vi "Read Show FP.vi"(8 "error in (no error)":errorcluster, 11 "Launch Functions Message in":refnum<class "Launch Functions Message.lvclass">) -> (0 "error out":errorcluster, 2 "Show FP?":bool, 3 "Launch Functions Message out":refnum<class "Launch Functions Message.lvclass">)   [LabVIEW 2016, in "Controller Actor.lvlib" / "Launch Functions Message.lvclass"]
uses:
  <userlib>/Common Components/Controller/Messages/Launch Functions Message/Launch Functions Message.lvclass
  <userlib>/Common Components/Controller/Messages/Launch Functions Message/Launch Functions Message.lvclass/Launch Functions Message.ctl
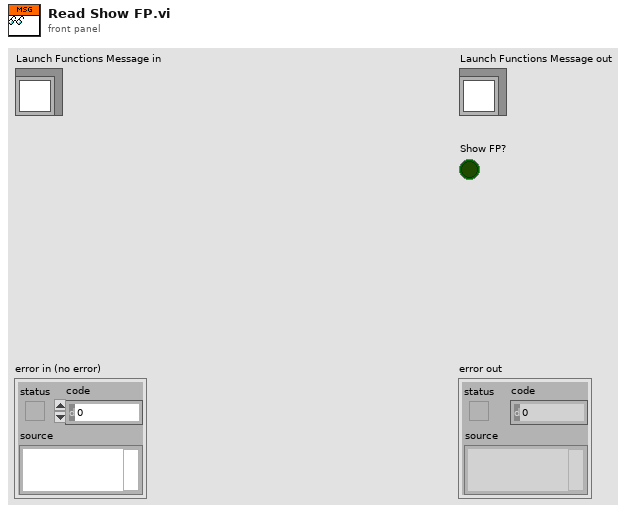
[diagram p1: front panel]
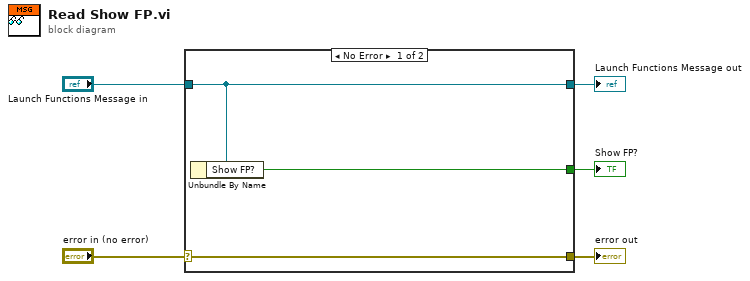
[diagram p0: block diagram]
diagram:
  n1 = case shown="No Error" "error in (no error)" {
    selector: "error in (no error)" -> [w8 w9]
    tunnel: [w8 w9] -> w4
    tunnel: [w7 w10] -> w2
    tunnel: "Launch Functions Message in" -> [w7 w10]
    tunnel: [w6 _] -> w1
    frame No Error {
      n2 = Unbundle By Name(w7) -> ("Show FP?"=w6:bool)
    }
    frame Error {
    }
  }
  "error out" <- w4
  "Launch Functions Message out" <- w2
  "Show FP?" <- w1
